vi "PH_BeamlineController.ProcCases.vi"(0 "i ref in":refnum<vi>, 1 "selector":string, 2 "Data":T1, 3 "call cluster":T2={"Object"="", "Selector"="", "CallType"=enum."synchronous", "Async Object"="", "Async Selector"="", "Data Descriptor"="", "Data"=[], "Error #"=0, "Expire"=0}, 5 "error in (no error)":errorcluster) -> (14 "i ref out":refnum<vi>, 17 "answer cluster":T2={"Object"="", "Selector"="", "CallType"=enum."synchronous", "Async Object"="", "Async Selector"="", "Data Descriptor"="", "Data"=[], "Error #"=0, "Expire"=0}, 19 "error out":errorcluster)   [LabVIEW 2014, in "PH_BeamlineController.lvlib"]
doc: "This method is called by a process from within the default case in the event loop. The methods of a class that are linked to events will be called from THIS method. Add your code here."
uses:
  PH_BeamlineController.lvlib
  CS_Core/CSSystem/CoreDefs/CoreDefs.call_type.ctl
  CS_Core/BaseProcess/BaseProcess.descriptor string definition.ctl
  CS_Core/CSSystem/CoreDefs/CoreDefs.rawDataType.ctl
  PH_Basics/PH_SystemInformation/PH_SystemInformationEnabling State.ctl
  PH_BeamlineController.Sources.ctl
  PH_BeamlineController.Targets.ctl
  PH_BeamlineController.PA DP Targets.ctl
  CS_Core/CSSystem/CoreLib/CoreLib.string 2 byte array.vi
  CS_Core/CSSystem/CoreLib/CoreLib.byte array 2 short.vi
  CS_Core/BaseProcess/BaseProcess.lvlib
  CS_Core/CAEObj/CAEObj.lvlib
  CS_Core/CSSystem/CoreLib/CoreLib.lvlib
  PH_Basics/PH_Common/PH_Common.lvlib
  PH_Basics/PH_StatusHandler/PH_StatusHandler.lvlib
  PH_BeamlineInformation/PH_BeamlineInformation.lvlib
  PH_Basics/PH_SystemInformation/PH_SystemInformation.lvlib
  CS_Core/CSSystem/CSSystemLib/CSSystemLib.lvlib
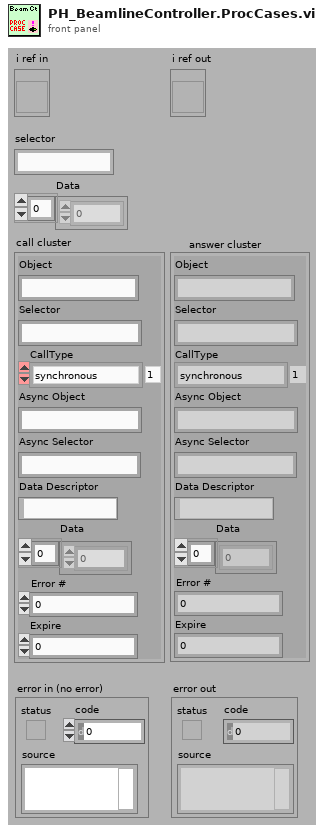
[diagram p1: front panel]
types:
  T1 = typedef "CoreDefs.rawDataType.ctl" = i8[]
  T2 = typedef "CoreDefs.call_type.ctl" = cluster{"Object":string, "Selector":string, "CallType":enum16{"simple", "synchronous", "asynchronous"}, "Async Object":string, "Async Selector":string, "Data Descriptor":T3, "Data":T1, "Error #":i32, "Expire":u32}
  T3 = typedef "BaseProcess.lvlib/BaseProcess.descriptor string definition.ctl" = string
  T4 = typedef "PH_SystemInformation.lvlib/PH_SystemInformationEnabling State.ctl" = i32
  T5 = cluster{"Enabling State":T4, "Enabling State":T4}
  T6 = typedef "PH_BeamlineController.lvlib/PH_BeamlineController.Sources.ctl" = enum16{"None", "YLF", "fs-Frontend", "ns-Frontend", "YLF and ns-Frontend", "fs- and ns-Frontend"}
  T7 = typedef "PH_BeamlineController.lvlib/PH_BeamlineController.Targets.ctl" = enum16{"None", "PreAmp", "Dump Exp Laserlab", "Exp Laserlab", "Calorimeter", "Dump Exp Laserbay", "Exp Laserbay", "Dump Exp Z6", "Exp Z6"}
  T8 = typedef "PH_BeamlineController.lvlib/PH_BeamlineController.PA DP Targets.ctl" = enum16{"None", "Dump PA Delayed Beam", "Dump PA Undelayed Beam", "Dumps PA Delayed and Undelayed Beam"}
  T9 = typedef "PH_BeamlineController.lvlib/PH_BeamlineController.i attribute.ctl" = cluster{"Vacuum Exp LB":cluster{"Channel":string, "Limit [mbar]":dbl, "Pressure [mbar]":dbl, "GUI Ref":refnum<vi>}, "Sources":T10[], "PA DP Targets":T11[], "Path":cluster{"Source":T6, "PA DP Target":T8, "Target":T7}, "Targets":cluster{"Name":T7, "GUI Ref":refnum<vi>, "Current State":bool, "Wanted State":bool, "Enabled":bool}[], "Status Tags":cluster{"Name":string, "Status":T12}[], "special GUI Refs":T13}
  T10 = typedef "PH_BeamlineController.lvlib/PH_BeamlineController.Source Attributes.ctl" = cluster{"Name":T6, "GUI Ref":refnum<vi>, "Current State":bool, "Wanted State":bool}
  T11 = typedef "PH_BeamlineController.lvlib/PH_BeamlineController.PA DP Target Attributes.ctl" = cluster{"Name":T8, "GUI Ref":refnum<vi>, "Current State":bool, "Wanted State":bool, "Enabled":bool}
  T12 = typedef "PH_StatusHandler.lvlib/PH_StatusHandler.Status.ctl" = i16
  T13 = typedef "PH_BeamlineController.lvlib/PH_BeamlineController.special GUI Refs.ctl" = cluster{"PA-Backreflection-Meas":refnum<vi>, "fs_Synchrolock_Watch":refnum<vi>}
  T14 = enum16{"Laser", "PreAmp", "MainAmp", "Exp 1", "Exp 2", "Exp 3", "Exp 4"}
  T15 = typedef "PH_BeamlineController.lvlib/PH_BeamlineController.Target Attributes.ctl" = cluster{"Name":T7, "GUI Ref":refnum<vi>, "Current State":bool, "Wanted State":bool, "Enabled":bool}
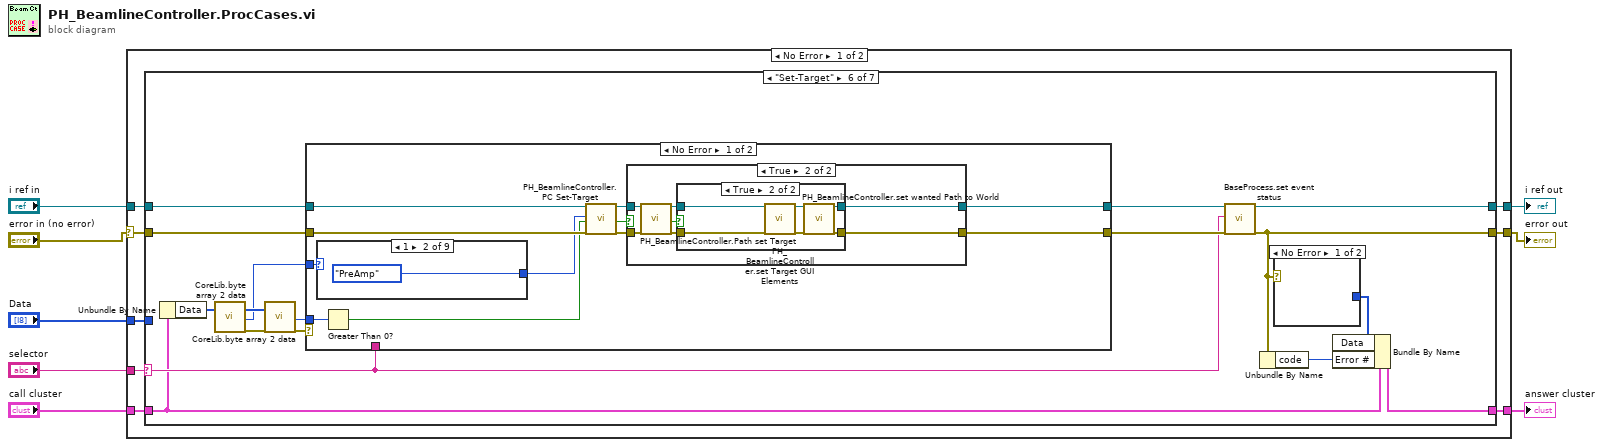
[diagram p0: block diagram]
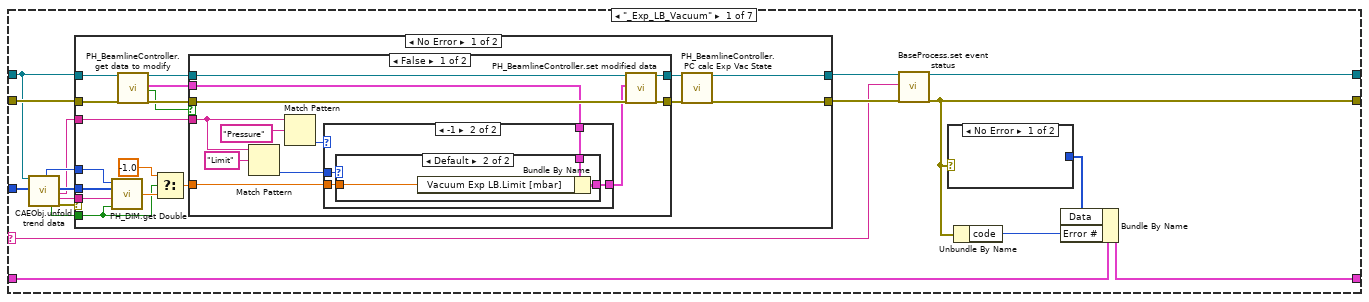
[diagram p2: hidden frame]
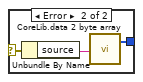
[diagram p3: hidden frame]
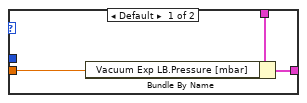
[diagram p4: hidden frame]
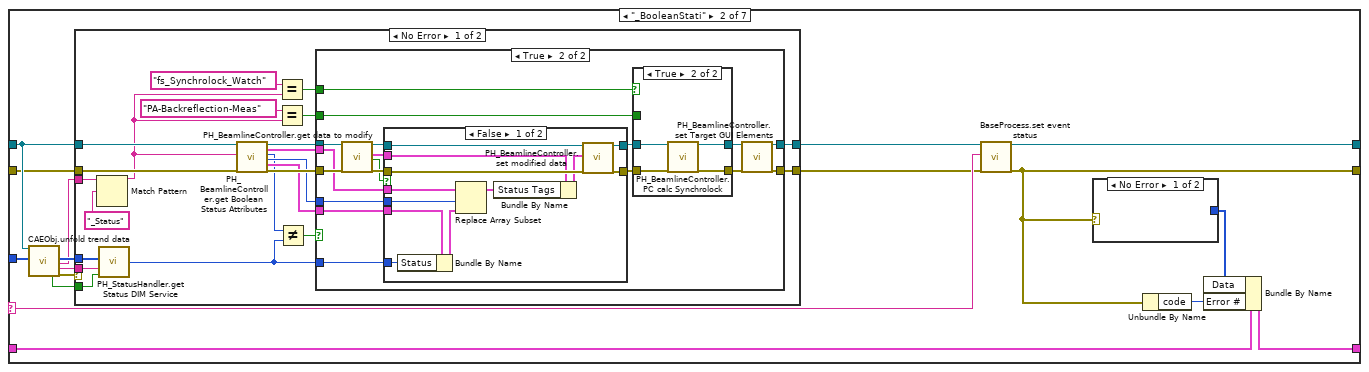
[diagram p8: hidden frame]
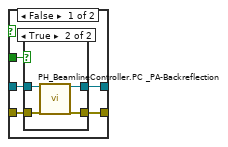
[diagram p10: hidden frame]
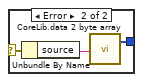
[diagram p14: hidden frame]
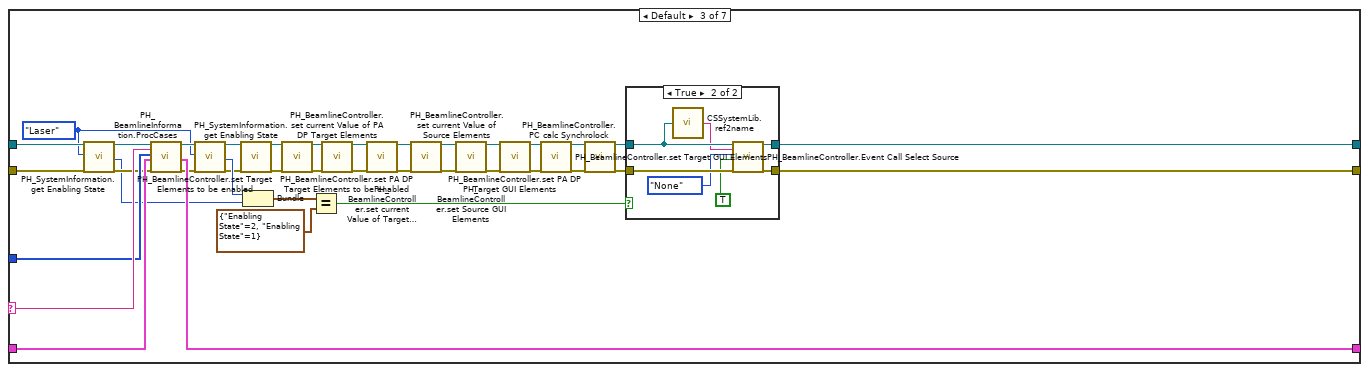
[diagram p15: hidden frame]
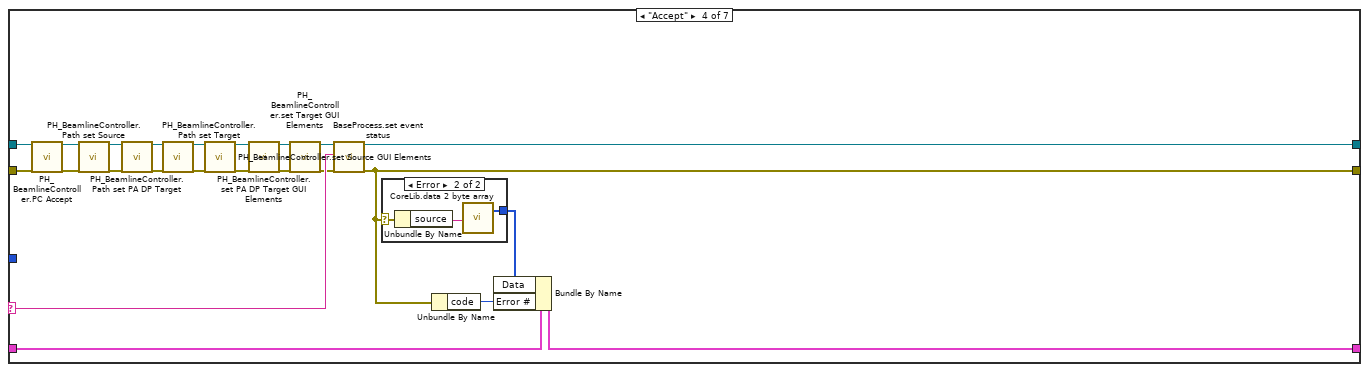
[diagram p17: hidden frame]
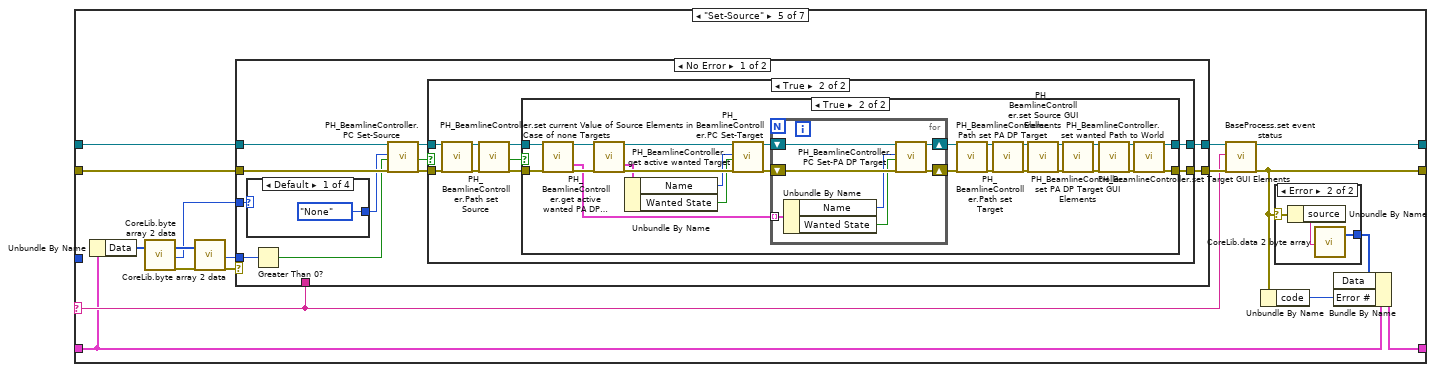
[diagram p19: hidden frame]
diagram:
  n1 = case shown="No Error" "error in (no error)" {
    selector: "error in (no error)" -> [w9 w463]
    tunnel: "selector" -> [w16 _]
    tunnel: [w15 w461] -> w7
    tunnel: "call cluster" -> [w14 w461]
    tunnel: "i ref in" -> [w13 w462]
    tunnel: [w12 w462] -> w4
    tunnel: [w11 w463] -> w3
    tunnel: "Data" -> [w10 _]
    frame No Error {
      n2 = case shown="\"Set-Target\"" w16 {
        selector: w16 -> [w19 w95 w210 w233 w252 w337 w398]
        tunnel: w13 -> [w33 w91 w191 w244 w255 w340 w401]
        tunnel: [w20 w97 w177 w238 w254 w339 w400] -> w12
        tunnel: w14 -> [w18 w93 w211 w234 w249 w334 w395]
        tunnel: [w17 w94 w212 w237 w250 w335 w396] -> w15
        tunnel: w9 -> [w34 w89 w213 w245 w253 w338 w399]
        tunnel: [w21 w96 w176 w236 w251 w336 w397] -> w11
        tunnel: w10 -> [w32 w92 w209 _ _ _ _]
        frame "_Exp_LB_Vacuum" {
          n3 = call "CAEObj.unfold trend data.vi"("i ref in"=w33, "raw trend data"=w32) -> ("quality"=w28:i32, "no link"=w27:bool, "data"=w29:i8[], "serviceName"=w26:string, "typeDescriptor"=w30:string, "error out"=w31:errorcluster)  [unwired: 9 in, 3 out]
          n4 = case shown="No Error" w31 {
            tunnel: [w48 w82] -> w22
            tunnel: w33 -> [w55 w82]
            tunnel: w34 -> [w54 w81]
            tunnel: [w49 w81] -> w23
            tunnel: w30 -> [w52 _]
            tunnel: w29 -> [w51 _]
            tunnel: w28 -> [w50 _]
            tunnel: w27 -> [w40 _]
            tunnel: w26 -> [w43 _]
            frame No Error {
              n5 = call "PH_DIM.get Double.vi"("no link"=w40, "typeDescriptor"=w52, "data"=w51, "quality"=w50) -> ("Value"=w41:dbl)
              n6 = call "PH_BeamlineController.get data to modify.vi"("i ref in"=w55, "error in (no error)"=w54) -> ("i ref out"=w46:refnum<vi>, "i attribute"=w42:T9, "timed out"=w44:bool, "error out"=w53:errorcluster)  [unwired: 14 in]
              n7 = Select(t=-1.0, s=w40, f=w41) -> (s? t:f=w38:dbl)
              n8 = case shown="False" w44 {
                tunnel: w53 -> [w67 w79]
                tunnel: [w66 w79] -> w47
                tunnel: w46 -> [w65 w80]
                tunnel: [w64 w80] -> w45
                tunnel: w43 -> [w58 _]
                tunnel: w42 -> [w62 _]
                tunnel: w38 -> [w59 _]
                frame False {
                  n9 = Match Pattern(string=w58, regular expression="Limit") -> (offset past match=w56:i32)  [unwired: 1 in, 3 out]
                  n10 = Match Pattern(string=w58, regular expression="Pressure") -> (offset past match=w61:i32)  [unwired: 1 in, 3 out]
                  n11 = case shown="-1" w61 {
                    tunnel: w62 -> [w70 w74]
                    tunnel: [w69 w73] -> w60
                    tunnel: w59 -> [w68 w72]
                    tunnel: w56 -> [_ w71]
                    frame Default {
                      n12 = Bundle By Name(cluster=w70, "Vacuum Exp LB.Pressure [mbar]"=w68) -> (w69:T9)
                    }
                    frame -1 {
                      n13 = case shown="Default" w71 {
                        tunnel: w74 -> [w75 w78]
                        tunnel: [w75 w77] -> w73
                        tunnel: w72 -> [_ w76]
                        frame 0 {
                        }
                        frame Default {
                          n14 = Bundle By Name(cluster=w78, "Vacuum Exp LB.Limit [mbar]"=w76) -> (w77:T9)
                        }
                      }
                    }
                  }
                  n15 = call "PH_BeamlineController.set modified data.vi"("i ref in"=w65, "i attribute"=w60, "error in (no error)"=w67) -> ("i ref out"=w64:refnum<vi>, "error out"=w66:errorcluster)  [unwired: 15 in]
                }
                frame True {
                }
              }
              n16 = call "PH_BeamlineController.PC calc Exp Vac State.vi"("i ref in"=w45, "error in"=w47) -> ("i ref out"=w48:refnum<vi>, "error out"=w49:errorcluster)  [unwired: 16 in]
            }
            frame Error {
            }
          }
          n17 = call "BaseProcess.set event status.vi"("i ref in"=w22, "EventStatus"=w19, "error in (no error)"=w23) -> ("i ref out"=w20:refnum<vi>, "error out"=w21:errorcluster)  [unwired: 14 in, 1 out]
          n18 = case shown="No Error" w21 {
            selector: w21 -> [_ w37]
            tunnel: [_ w35] -> w24
            frame No Error {
            }
            frame Error {
              n19 = Unbundle By Name(w37) -> ("source"=w36:string)
              n20 = call-poly "CoreLib.data 2 byte array.vi"("string"=w36) -> ("byteArray out"=w35:T1)  [unwired: 18 in]
            }
          }
          n21 = Unbundle By Name(w21) -> ("code"=w25:i32)
          n22 = Bundle By Name(cluster=w18, "Data"=w24, "Error #"=w25) -> (w17:T2)
        }
        frame "_BooleanStati" {
          n23 = call "CAEObj.unfold trend data.vi"("i ref in"=w91, "raw trend data"=w92) -> ("no link"=w84:bool, "data"=w87:i8[], "serviceName"=w83:string, "typeDescriptor"=w85:string, "error out"=w86:errorcluster)  [unwired: 9 in, 4 out]
          n24 = case shown="No Error" w86 {
            tunnel: [w118 w172] -> w90
            tunnel: w91 -> [w114 w172]
            tunnel: w89 -> [w112 w171]
            tunnel: [w117 w171] -> w88
            tunnel: w84 -> [w119 _]
            tunnel: w87 -> [w121 _]
            tunnel: w85 -> [w120 _]
            tunnel: w83 -> [w116 _]
            frame No Error {
              n25 = Match Pattern(string=w116, regular expression="_Status") -> (before substring=w102:string)  [unwired: 1 in, 3 out]
              n26 = call "PH_StatusHandler.get Status DIM Service.vi"("no link"=w119, "typeDescriptor"=w120, "data"=w121) -> ("Status"=w106:T12)  [unwired: 1 in]
              n27 = call "PH_BeamlineController.get Boolean Status Attributes.vi"("VI in"=w114, "Name"=w102, "error in (no error)"=w112) -> ("VI out"=w113:refnum<vi>, "Status Tags"=w110:cluster{"Name":string, "Status":T12}[], "Status"=w107:T12, "index of element"=w108:i32, "Tag"=w109:cluster{"Name":string, "Status":T12}, "error out"=w111:errorcluster)  [unwired: 11 in]
              n28 = Equal?(x="fs_Synchrolock_Watch" ("Synchrolock.Instance"), y=w102) -> (x = y?=w103:bool)
              n29 = Equal?(x="PA-Backreflection-Meas" ("Instance PA Backreflection"), y=w102) -> (x = y?=w100:bool)
              n30 = Not Equal?(x=w107, y=w106) -> (x != y?=w105:bool)
              n31 = case shown="True" w105 {
                tunnel: w106 -> [_ w137]
                tunnel: [w123 w127] -> w118
                tunnel: [w122 w126] -> w117
                tunnel: w113 -> [w123 w136]
                tunnel: w111 -> [w122 w135]
                tunnel: w110 -> [_ w134]
                tunnel: w109 -> [_ w133]
                tunnel: w108 -> [_ w132]
                tunnel: w103 -> [_ w129]
                tunnel: w100 -> [_ w128]
                frame False {
                }
                frame True {
                  n32 = call "PH_BeamlineController.get data to modify.vi"("i ref in"=w136, "error in (no error)"=w135) -> ("i ref out"=w140:refnum<vi>, "i attribute"=w138:T9, "timed out"=w139:bool, "error out"=w141:errorcluster)  [unwired: 14 in]
                  n33 = case shown="False" w139 {
                    tunnel: w141 -> [w168 w169]
                    tunnel: [w167 w169] -> w130
                    tunnel: w140 -> [w166 w170]
                    tunnel: [w165 w170] -> w131
                    tunnel: w138 -> [w164 _]
                    tunnel: w137 -> [w157 _]
                    tunnel: w134 -> [w161 _]
                    tunnel: w133 -> [w160 _]
                    tunnel: w132 -> [w159 _]
                    frame False {
                      n34 = Bundle By Name(cluster=w160, "Status"=w157) -> (w158:cluster{"Name":string, "Status":T12})
                      n35 = Replace Array Subset(array=w161, new element=w158, index=w159) -> (w162:cluster{"Name":string, "Status":T12}[])
                      n36 = Bundle By Name(cluster=w164, "Status Tags"=w162) -> (w163:T9)
                      n37 = call "PH_BeamlineController.set modified data.vi"("i ref in"=w166, "i attribute"=w163, "error in (no error)"=w168) -> ("i ref out"=w165:refnum<vi>, "error out"=w167:errorcluster)  [unwired: 15 in]
                    }
                    frame True {
                    }
                  }
                  n38 = case shown="True" w129 {
                    tunnel: [w144 w156] -> w125
                    tunnel: w131 -> [w146 w155]
                    tunnel: [w143 w154] -> w124
                    tunnel: w130 -> [w145 w153]
                    tunnel: w128 -> [w142 _]
                    frame False {
                      n39 = case shown="True" w142 {
                        tunnel: w146 -> [w148 w152]
                        tunnel: w145 -> [w147 w151]
                        tunnel: [w148 w150] -> w144
                        tunnel: [w147 w149] -> w143
                        frame False {
                        }
                        frame True {
                          n40 = call "PH_BeamlineController.PC _PA-Backreflection.vi"("i ref in"=w152, "error IO"=w151) -> ("i ref out"=w150:refnum<vi>, "error out"=w149:errorcluster)  [unwired: 16 in]
                        }
                      }
                    }
                    frame True {
                      n41 = call "PH_BeamlineController.PC calc Synchrolock.vi"("i ref in"=w155, "error in"=w153) -> ("i ref out"=w156:refnum<vi>, "error out"=w154:errorcluster)  [unwired: 16 in]
                    }
                  }
                  n42 = call "PH_BeamlineController.set Target GUI Elements.vi"("VI in"=w125, "error in (no error)"=w124) -> ("VI out"=w127:refnum<vi>, "error out"=w126:errorcluster)  [unwired: 16 in]
                }
              }
            }
            frame Error {
            }
          }
          n43 = call "BaseProcess.set event status.vi"("i ref in"=w90, "EventStatus"=w95, "error in (no error)"=w88) -> ("i ref out"=w97:refnum<vi>, "error out"=w96:errorcluster)  [unwired: 14 in, 1 out]
          n44 = case shown="No Error" w96 {
            selector: w96 -> [_ w175]
            tunnel: [_ w173] -> w98
            frame No Error {
            }
            frame Error {
              n45 = Unbundle By Name(w175) -> ("source"=w174:string)
              n46 = call-poly "CoreLib.data 2 byte array.vi"("string"=w174) -> ("byteArray out"=w173:T1)  [unwired: 18 in]
            }
          }
          n47 = Unbundle By Name(w96) -> ("code"=w99:i32)
          n48 = Bundle By Name(cluster=w93, "Data"=w98, "Error #"=w99) -> (w94:T2)
        }
        frame Default {
          w187 = T14."Laser" ("Wanted State")
          # "In the default case, always call the ProcCase method of the parent class"
          n49 = call "PH_SystemInformation.get Enabling State.vi"("i ref in"=w191, "Wanted State"=w187, "error in (no error)"=w213) -> ("i ref out"=w190:refnum<vi>, "Enabling State"=w186:T4, "error out"=w192:errorcluster)  [unwired: 14 in]
          n50 = call "PH_BeamlineInformation.ProcCases.vi"("i ref in"=w190, "selector"=w210, "Data"=w209, "call cluster"=w211, "error in (no error)"=w192) -> ("i ref out"=w189:refnum<vi>, "answer cluster"=w212:T2, "error out"=w188:errorcluster)  [unwired: 12 in]
          n51 = call "PH_SystemInformation.get Enabling State.vi"("i ref in"=w189, "Wanted State"=w187, "error in (no error)"=w188) -> ("i ref out"=w181:refnum<vi>, "Enabling State"=w185:T4, "error out"=w180:errorcluster)  [unwired: 14 in]
          n52 = call "PH_BeamlineController.set Target Elements to be enabled.vi"("VI in"=w181, "error in (no error)"=w180) -> ("VI out"=w206:refnum<vi>, "error out"=w207:errorcluster)  [unwired: 16 in]
          n53 = Bundle("Enabling State"=w185, "Enabling State"=w186) -> (w184:T5)  [unwired: 1 in]
          n54 = call "PH_BeamlineController.set PA DP Target Elements to be enabled.vi"("VI in"=w206, "error in (no error)"=w207) -> ("VI out"=w198:refnum<vi>, "error out"=w197:errorcluster)  [unwired: 16 in]
          n55 = Equal?(x=w184, y=T5 {"Enabling State"=2, "Enabling State"=1}) -> (x = y?=w182:bool)
          n56 = call "PH_BeamlineController.set current Value of PA DP Target Elements.vi"("VI in"=w198, "error in (no error)"=w197) -> ("VI out"=w202:refnum<vi>, "error out"=w201:errorcluster)  [unwired: 16 in]
          n57 = call "PH_BeamlineController.set current Value of Target Elements.vi"("VI in"=w202, "error in (no error)"=w201) -> ("VI out"=w195:refnum<vi>, "error out"=w196:errorcluster)  [unwired: 16 in]
          n58 = call "PH_BeamlineController.set current Value of Source Elements.vi"("VI in"=w195, "error in (no error)"=w196) -> ("VI out"=w194:refnum<vi>, "error out"=w193:errorcluster)  [unwired: 16 in]
          n59 = call "PH_BeamlineController.set Source GUI Elements.vi"("VI in"=w194, "error in (no error)"=w193) -> ("VI out"=w204:refnum<vi>, "error out"=w208:errorcluster)  [unwired: 16 in]
          n60 = call "PH_BeamlineController.set PA DP Target GUI Elements.vi"("VI in"=w204, "error in (no error)"=w208) -> ("VI out"=w203:refnum<vi>, "error out"=w205:errorcluster)  [unwired: 16 in]
          n61 = call "PH_BeamlineController.set Target GUI Elements.vi"("VI in"=w203, "error in (no error)"=w205) -> ("VI out"=w200:refnum<vi>, "error out"=w199:errorcluster)  [unwired: 16 in]
          n62 = call "PH_BeamlineController.PC calc Synchrolock.vi"("i ref in"=w200, "error in"=w199) -> ("i ref out"=w179:refnum<vi>, "error out"=w178:errorcluster)  [unwired: 16 in]
          n63 = case shown="True" w182 {
            tunnel: w178 -> [w214 w222]
            tunnel: w179 -> [w215 w217]
            tunnel: [w215 w220] -> w177
            tunnel: [w214 w219] -> w176
            frame False {
            }
            frame True {
              n64 = call "CSSystemLib.ref2name.vi"("obj refnum"=w217) -> ("name"=w216:string)
              n65 = call "PH_BeamlineController.Event Call Select Source.vi"("i ref in"=w217, "Instance"=w216, "Source"=PH_BeamlineController.Sources."None", "on(off"=TRUE, "error in (no error)"=w222) -> ("i ref out"=w220:refnum<vi>, "error out"=w219:errorcluster)  [unwired: 13 in]
            }
          }
        }
        frame "Accept" {
          # "In the default case, always call the ProcCase method of the parent class"
          n66 = call "PH_BeamlineController.PC Accept.vi"("i ref in"=w244, "error in (no error)"=w245) -> ("i ref out"=w228:refnum<vi>, "error out"=w224:errorcluster)  [unwired: 16 in]
          n67 = call "PH_BeamlineController.Path set Source.vi"("i ref in"=w228, "error in (no error)"=w224) -> ("i ref out"=w230:refnum<vi>, "error out"=w226:errorcluster)  [unwired: 15 in, 1 out]
          n68 = call "PH_BeamlineController.Path set PA DP Target.vi"("i ref in"=w230, "error in (no error)"=w226) -> ("i ref out"=w229:refnum<vi>, "error out"=w225:errorcluster)  [unwired: 15 in, 1 out]
          n69 = call "PH_BeamlineController.Path set Target.vi"("i ref in"=w229, "error in (no error)"=w225) -> ("i ref out"=w227:refnum<vi>, "error out"=w223:errorcluster)  [unwired: 15 in, 1 out]
          n70 = call "PH_BeamlineController.set Source GUI Elements.vi"("VI in"=w227, "error in (no error)"=w223) -> ("VI out"=w241:refnum<vi>, "error out"=w243:errorcluster)  [unwired: 16 in]
          n71 = call "PH_BeamlineController.set PA DP Target GUI Elements.vi"("VI in"=w241, "error in (no error)"=w243) -> ("VI out"=w240:refnum<vi>, "error out"=w242:errorcluster)  [unwired: 16 in]
          n72 = call "PH_BeamlineController.set Target GUI Elements.vi"("VI in"=w240, "error in (no error)"=w242) -> ("VI out"=w232:refnum<vi>, "error out"=w231:errorcluster)  [unwired: 16 in]
          n73 = call "BaseProcess.set event status.vi"("i ref in"=w232, "EventStatus"=w233, "error in (no error)"=w231) -> ("i ref out"=w238:refnum<vi>, "error out"=w236:errorcluster)  [unwired: 14 in, 1 out]
          n74 = case shown="Error" w236 {
            selector: w236 -> [_ w248]
            tunnel: [_ w246] -> w239
            frame No Error {
            }
            frame Error {
              n75 = Unbundle By Name(w248) -> ("source"=w247:string)
              n76 = call-poly "CoreLib.data 2 byte array.vi"("string"=w247) -> ("byteArray out"=w246:T1)  [unwired: 18 in]
            }
          }
          n77 = Unbundle By Name(w236) -> ("code"=w235:i32)
          n78 = Bundle By Name(cluster=w234, "Data"=w239, "Error #"=w235) -> (w237:T2)
        }
        frame "Set-Source" {
          # "In the default case, always call the ProcCase method of the parent class"
          n79 = Unbundle By Name(w249) -> ("Data"=w261:T1)
          n80 = call-poly "CoreLib.byte array 2 data.vi"("byteArray"=w261) -> ("byteArray out"=w259:T1, "i16"=w257:i16, "error out"=w260:errorcluster)  [unwired: 16 in]
          n81 = call-poly "CoreLib.byte array 2 data.vi"("byteArray"=w259, "error in (no error)"=w260) -> ("i16"=w256:i16, "error out"=w258:errorcluster)  [unwired: 15 in, 1 out]
          n82 = case shown="No Error" w258 {
            tunnel: [w270 w333] -> w262
            tunnel: w255 -> [w279 w333]
            tunnel: w253 -> [w278 w332]
            tunnel: [w272 w331] -> w263
            tunnel: w252 -> [_ w330]
            tunnel: w257 -> [w273 _]
            tunnel: w256 -> [w277 _]
            frame No Error {
              n83 = case shown="Default" w273 {
                tunnel: [PH_BeamlineController.Sources."None" ("Source") PH_BeamlineController.Sources."YLF" ("Source") PH_BeamlineController.Sources."fs-Frontend" ("Source") PH_BeamlineController.Sources."ns-Frontend" ("Source")] -> w274
                frame Default {
                }
                frame 1 {
                }
                frame 2 {
                }
                frame 3 {
                }
              }
              n84 = Greater Than 0?(x=w277) -> (x > 0?=w276:bool)
              n85 = call "PH_BeamlineController.PC Set-Source.vi"("i ref in"=w279, "Source"=w274, "Value"=w276, "error in (no error)"=w278) -> ("i ref out"=w271:refnum<vi>, "Sources changed?"=w269:bool, "error out"=w275:errorcluster)  [unwired: 13 in]
              n86 = case shown="True" w269 {
                tunnel: w275 -> [w280 w285]
                tunnel: [w280 w289] -> w272
                tunnel: w271 -> [w281 w284]
                tunnel: [w281 w287] -> w270
                frame False {
                }
                frame True {
                  n87 = call "PH_BeamlineController.set current Value of Source Elements in Case of none Targets.vi"("VI in"=w284, "error in (no error)"=w285) -> ("VI out"=w283:refnum<vi>, "error out"=w282:errorcluster)  [unwired: 16 in]
                  n88 = call "PH_BeamlineController.Path set Source.vi"("i ref in"=w283, "error in (no error)"=w282) -> ("i ref out"=w288:refnum<vi>, "Path changed?"=w286:bool, "error out"=w290:errorcluster)  [unwired: 15 in]
                  n89 = case shown="True" w286 {
                    tunnel: w290 -> [w291 w309]
                    tunnel: [w291 w314] -> w289
                    tunnel: w288 -> [w292 w302]
                    tunnel: [w292 w312] -> w287
                    frame False {
                    }
                    frame True {
                      n90 = call "PH_BeamlineController.get active wanted PA DP Targets.vi"("VI in"=w302, "error in (no error)"=w309) -> ("VI out"=w301:refnum<vi>, "active wanted State PA DP Targets Attributes"=w299:T11[], "error out"=w300:errorcluster)  [unwired: 15 in]
                      n91 = call "PH_BeamlineController.get active wanted Target.vi"("VI in"=w301, "error in (no error)"=w300) -> ("VI out"=w310:refnum<vi>, "active wanted State Target Attributes"=w307:T15, "error out"=w308:errorcluster)  [unwired: 14 in, 1 out]
                      n92 = Unbundle By Name(w307) -> ("Name"=w306:T7, "Wanted State"=w305:bool)
                      n93 = call "PH_BeamlineController.PC Set-Target.vi"("i ref in"=w310, "Targets"=w306, "Value"=w305, "error in (no error)"=w308) -> ("i ref out"=w303:refnum<vi>, "error out"=w311:errorcluster)  [unwired: 13 in, 1 out]
                      n94 = for {
                        tunnel: w299 -> [w322] mode=indexing
                        shift-right: [w324] -> w304
                        shift-left: w311 -> [w325]
                        shift-right: [w319] -> w297
                        shift-left: w303 -> [w323]
                        n95 = Unbundle By Name(w322) -> ("Name"=w321:T8, "Wanted State"=w320:bool)
                        n96 = call "PH_BeamlineController.PC Set-PA DP Target.vi"("i ref in"=w323, "PA DP Targets"=w321, "Value"=w320, "error in (no error)"=w325) -> ("i ref out"=w319:refnum<vi>, "error out"=w324:errorcluster)  [unwired: 13 in, 1 out]
                      }
                      n97 = call "PH_BeamlineController.Path set PA DP Target.vi"("i ref in"=w297, "error in (no error)"=w304) -> ("i ref out"=w296:refnum<vi>, "error out"=w298:errorcluster)  [unwired: 15 in, 1 out]
                      n98 = call "PH_BeamlineController.Path set Target.vi"("i ref in"=w296, "error in (no error)"=w298) -> ("i ref out"=w316:refnum<vi>, "error out"=w317:errorcluster)  [unwired: 15 in, 1 out]
                      n99 = call "PH_BeamlineController.set Source GUI Elements.vi"("VI in"=w316, "error in (no error)"=w317) -> ("VI out"=w294:refnum<vi>, "error out"=w318:errorcluster)  [unwired: 16 in]
                      n100 = call "PH_BeamlineController.set PA DP Target GUI Elements.vi"("VI in"=w294, "error in (no error)"=w318) -> ("VI out"=w293:refnum<vi>, "error out"=w295:errorcluster)  [unwired: 16 in]
                      n101 = call "PH_BeamlineController.set Target GUI Elements.vi"("VI in"=w293, "error in (no error)"=w295) -> ("VI out"=w313:refnum<vi>, "error out"=w315:errorcluster)  [unwired: 16 in]
                      n102 = call "PH_BeamlineController.set wanted Path to World.vi"("VI in"=w313, "error in (no error)"=w315) -> ("VI out"=w312:refnum<vi>, "error out"=w314:errorcluster)  [unwired: 16 in]
                    }
                  }
                }
              }
            }
            frame Error {
              n103 = call "CoreLib.set data type mismatch.vi"("error in (no error)"=w332, "error source"=w330) -> ("error out"=w331:errorcluster)  [unwired: 17 in]
            }
          }
          n104 = call "BaseProcess.set event status.vi"("i ref in"=w262, "EventStatus"=w252, "error in (no error)"=w263) -> ("i ref out"=w254:refnum<vi>, "error out"=w251:errorcluster)  [unwired: 14 in, 1 out]
          n105 = Unbundle By Name(w251) -> ("code"=w265:i32)
          n106 = case shown="Error" w251 {
            selector: w251 -> [_ w268]
            tunnel: [_ w266] -> w264
            frame No Error {
            }
            frame Error {
              n107 = Unbundle By Name(w268) -> ("source"=w267:string)
              n108 = call-poly "CoreLib.data 2 byte array.vi"("string"=w267) -> ("byteArray out"=w266:T1)  [unwired: 18 in]
            }
          }
          n109 = Bundle By Name(cluster=w249, "Data"=w264, "Error #"=w265) -> (w250:T2)
        }
        frame "Set-Target" {
          # "In the default case, always call the ProcCase method of the parent class"
          n110 = Unbundle By Name(w334) -> ("Data"=w346:T1)
          n111 = call-poly "CoreLib.byte array 2 data.vi"("byteArray"=w346) -> ("byteArray out"=w344:T1, "i16"=w342:i16, "error out"=w345:errorcluster)  [unwired: 16 in]
          n112 = call-poly "CoreLib.byte array 2 data.vi"("byteArray"=w344, "error in (no error)"=w345) -> ("i16"=w341:i16, "error out"=w343:errorcluster)  [unwired: 15 in, 1 out]
          n113 = case shown="No Error" w343 {
            tunnel: [w355 w394] -> w347
            tunnel: w340 -> [w364 w394]
            tunnel: w338 -> [w363 w393]
            tunnel: [w357 w392] -> w348
            tunnel: w337 -> [_ w391]
            tunnel: w342 -> [w358 _]
            tunnel: w341 -> [w362 _]
            frame No Error {
              n114 = case shown="1" w358 {
                tunnel: [PH_BeamlineController.Targets."None" ("Targets") PH_BeamlineController.Targets."PreAmp" ("Targets") PH_BeamlineController.Targets."Dump Exp Laserlab" ("Targets") PH_BeamlineController.Targets."Exp Laserlab" ("Targets") PH_BeamlineController.Targets."Calorimeter" ("Targets") PH_BeamlineController.Targets."Dump Exp Laserbay" ("Targets") PH_BeamlineController.Targets."Exp Laserbay" ("Targets") PH_BeamlineController.Targets."Dump Exp Z6" ("Targets") PH_BeamlineController.Targets."Exp Z6" ("Targets")] -> w359
                frame Default {
                }
                frame 1 {
                }
                frame 2 {
                }
                frame 3 {
                }
                frame 4 {
                }
                frame 5 {
                }
                frame 6 {
                }
                frame 7 {
                }
                frame 8 {
                }
              }
              n115 = Greater Than 0?(x=w362) -> (x > 0?=w361:bool)
              n116 = call "PH_BeamlineController.PC Set-Target.vi"("i ref in"=w364, "Targets"=w359, "Value"=w361, "error in (no error)"=w363) -> ("i ref out"=w356:refnum<vi>, "Targets changed?"=w354:bool, "error out"=w360:errorcluster)  [unwired: 13 in]
              n117 = case shown="True" w354 {
                tunnel: w360 -> [w365 w373]
                tunnel: [w365 w370] -> w357
                tunnel: w356 -> [w366 w371]
                tunnel: [w366 w368] -> w355
                frame False {
                }
                frame True {
                  n118 = call "PH_BeamlineController.Path set Target.vi"("i ref in"=w371, "error in (no error)"=w373) -> ("i ref out"=w369:refnum<vi>, "Path changed?"=w367:bool, "error out"=w372:errorcluster)  [unwired: 15 in]
                  n119 = case shown="True" w367 {
                    tunnel: w372 -> [w374 w376]
                    tunnel: [w374 w380] -> w370
                    tunnel: w369 -> [w375 w377]
                    tunnel: [w375 w378] -> w368
                    frame False {
                    }
                    frame True {
                      n120 = call "PH_BeamlineController.set Target GUI Elements.vi"("VI in"=w377, "error in (no error)"=w376) -> ("VI out"=w379:refnum<vi>, "error out"=w381:errorcluster)  [unwired: 16 in]
                      n121 = call "PH_BeamlineController.set wanted Path to World.vi"("VI in"=w379, "error in (no error)"=w381) -> ("VI out"=w378:refnum<vi>, "error out"=w380:errorcluster)  [unwired: 16 in]
                    }
                  }
                }
              }
            }
            frame Error {
              n122 = call "CoreLib.set data type mismatch.vi"("error in (no error)"=w393, "error source"=w391) -> ("error out"=w392:errorcluster)  [unwired: 17 in]
            }
          }
          n123 = call "BaseProcess.set event status.vi"("i ref in"=w347, "EventStatus"=w337, "error in (no error)"=w348) -> ("i ref out"=w339:refnum<vi>, "error out"=w336:errorcluster)  [unwired: 14 in, 1 out]
          n124 = Unbundle By Name(w336) -> ("code"=w350:i32)
          n125 = case shown="No Error" w336 {
            selector: w336 -> [_ w353]
            tunnel: [_ w351] -> w349
            frame No Error {
            }
            frame Error {
              n126 = Unbundle By Name(w353) -> ("source"=w352:string)
              n127 = call-poly "CoreLib.data 2 byte array.vi"("string"=w352) -> ("byteArray out"=w351:T1)  [unwired: 18 in]
            }
          }
          n128 = Bundle By Name(cluster=w334, "Data"=w349, "Error #"=w350) -> (w335:T2)
        }
        frame "Set-PADPTarget" {
          # "In the default case, always call the ProcCase method of the parent class"
          n129 = Unbundle By Name(w395) -> ("Data"=w407:T1)
          n130 = call-poly "CoreLib.byte array 2 data.vi"("byteArray"=w407) -> ("byteArray out"=w405:T1, "i16"=w403:i16, "error out"=w406:errorcluster)  [unwired: 16 in]
          n131 = call-poly "CoreLib.byte array 2 data.vi"("byteArray"=w405, "error in (no error)"=w406) -> ("i16"=w402:i16, "error out"=w404:errorcluster)  [unwired: 15 in, 1 out]
          n132 = case shown="No Error" w404 {
            tunnel: [w416 w460] -> w408
            tunnel: w401 -> [w425 w460]
            tunnel: w399 -> [w424 w459]
            tunnel: [w418 w458] -> w409
            tunnel: w398 -> [_ w457]
            tunnel: w403 -> [w419 _]
            tunnel: w402 -> [w423 _]
            frame No Error {
              n133 = case shown="2" w419 {
                tunnel: [PH_BeamlineController.PA_DP_Targets."None" ("Targets") PH_BeamlineController.PA_DP_Targets."Dump PA Delayed Beam" ("Targets") PH_BeamlineController.PA_DP_Targets."Dump PA Undelayed Beam" ("Targets")] -> w420
                frame Default {
                }
                frame 1 {
                }
                frame 2 {
                }
              }
              n134 = Greater Than 0?(x=w423) -> (x > 0?=w422:bool)
              n135 = call "PH_BeamlineController.PC Set-PA DP Target.vi"("i ref in"=w425, "PA DP Targets"=w420, "Value"=w422, "error in (no error)"=w424) -> ("i ref out"=w417:refnum<vi>, "PA DP Targets changed?"=w415:bool, "error out"=w421:errorcluster)  [unwired: 13 in]
              n136 = case shown="True" w415 {
                tunnel: w421 -> [w426 w434]
                tunnel: [w426 w431] -> w418
                tunnel: w417 -> [w427 w432]
                tunnel: [w427 w429] -> w416
                frame False {
                }
                frame True {
                  n137 = call "PH_BeamlineController.Path set PA DP Target.vi"("i ref in"=w432, "error in (no error)"=w434) -> ("i ref out"=w430:refnum<vi>, "Path changed?"=w428:bool, "error out"=w433:errorcluster)  [unwired: 15 in]
                  n138 = case shown="True" w428 {
                    tunnel: w433 -> [w435 w438]
                    tunnel: [w435 w452] -> w431
                    tunnel: w430 -> [w436 w440]
                    tunnel: [w436 w450] -> w429
                    frame False {
                    }
                    frame True {
                      n139 = call "PH_BeamlineController.get active wanted Target.vi"("VI in"=w440, "error in (no error)"=w438) -> ("VI out"=w441:refnum<vi>, "active wanted State Target Attributes"=w443:T15, "error out"=w442:errorcluster)  [unwired: 14 in, 1 out]
                      n140 = Unbundle By Name(w443) -> ("Name"=w444:T7, "Wanted State"=w445:bool)
                      n141 = call "PH_BeamlineController.PC Set-Target.vi"("i ref in"=w441, "Targets"=w444, "Value"=w445, "error in (no error)"=w442) -> ("i ref out"=w446:refnum<vi>, "error out"=w447:errorcluster)  [unwired: 13 in, 1 out]
                      n142 = call "PH_BeamlineController.Path set Target.vi"("i ref in"=w446, "error in (no error)"=w447) -> ("i ref out"=w448:refnum<vi>, "error out"=w449:errorcluster)  [unwired: 15 in, 1 out]
                      n143 = call "PH_BeamlineController.set Target GUI Elements.vi"("VI in"=w448, "error in (no error)"=w449) -> ("VI out"=w439:refnum<vi>, "error out"=w437:errorcluster)  [unwired: 16 in]
                      n144 = call "PH_BeamlineController.set PA DP Target GUI Elements.vi"("VI in"=w439, "error in (no error)"=w437) -> ("VI out"=w451:refnum<vi>, "error out"=w453:errorcluster)  [unwired: 16 in]
                      n145 = call "PH_BeamlineController.set wanted Path to World.vi"("VI in"=w451, "error in (no error)"=w453) -> ("VI out"=w450:refnum<vi>, "error out"=w452:errorcluster)  [unwired: 16 in]
                    }
                  }
                }
              }
            }
            frame Error {
              n146 = call "CoreLib.set data type mismatch.vi"("error in (no error)"=w459, "error source"=w457) -> ("error out"=w458:errorcluster)  [unwired: 17 in]
            }
          }
          n147 = call "BaseProcess.set event status.vi"("i ref in"=w408, "EventStatus"=w398, "error in (no error)"=w409) -> ("i ref out"=w400:refnum<vi>, "error out"=w397:errorcluster)  [unwired: 14 in, 1 out]
          n148 = Unbundle By Name(w397) -> ("code"=w411:i32)
          n149 = case shown="Error" w397 {
            selector: w397 -> [_ w414]
            tunnel: [_ w412] -> w410
            frame No Error {
            }
            frame Error {
              n150 = Unbundle By Name(w414) -> ("source"=w413:string)
              n151 = call-poly "CoreLib.data 2 byte array.vi"("string"=w413) -> ("byteArray out"=w412:T1)  [unwired: 18 in]
            }
          }
          n152 = Bundle By Name(cluster=w395, "Data"=w410, "Error #"=w411) -> (w396:T2)
        }
      }
    }
    frame Error {
    }
  }
  "answer cluster" <- w7
  "i ref out" <- w4
  "error out" <- w3
